vi "WFS Average Image Rolling.vi"(8 "error in (no error)":errorcluster {"code" format="%.0x"}, 9 "Reset":i32 format="%.0g", 10 "Average Count":i32 format="%.0g", 11 "instrument handle":refnum<visa-resource-name>) -> (0 "error out":errorcluster {"code" format="%.0x"}, 3 "instrument handle out":refnum<visa-resource-name>)   [LabVIEW 2020]
doc: "This VI generates a rolling averaged image based on all previously entered camera images in ImageBuf. The VI returns after each call and the averaged image is returned in ImageBuf and also stored in ImageBufAveraged.\n\nThe new rolling averaged image is calculated pixel by pixel according to the formula:\n(AverageCount - 1) * ImageBufAvg + ImageBuf) / AverageCount\n\nNote:\nAs soon as the image size is changed by VI ConfigureCam the averaging process is re-started.\nThis VI is not available in Highspeed Mode!"
uses:
  WFS_32.dll
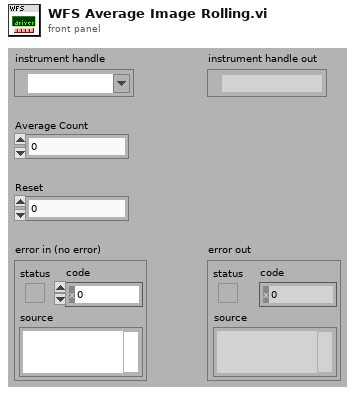
[diagram p1: front panel]
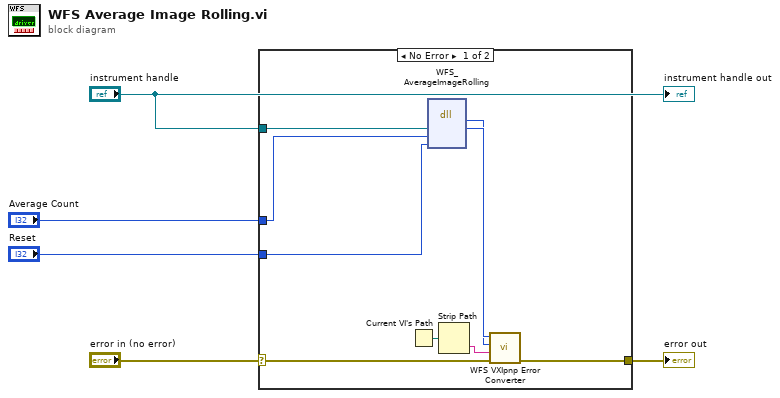
[diagram p0: block diagram]
diagram:
  n1 = case shown="No Error" "error in (no error)" {
    selector: "error in (no error)" -> [w9 w15]
    tunnel: [w8 w15] -> w5
    tunnel: "instrument handle" -> [w13 _]
    tunnel: "Average Count" -> [w7 _]
    tunnel: "Reset" -> [w6 _]
    frame No Error {
      n2 = Current VI's Path() -> (path=w14:path)
      n3 = dll-call lib="WFS_*.*" fn="WFS_AverageImageRolling"("Instrument Handle"=w13, "Average Count"=w7, "Reset"=w6) -> (w11:i32, "Instrument Handle"=w12:u32)  [unwired: 5 in, 2 out]
      n4 = Strip Path(path=w14) -> (name=w10:string)  [unwired: 1 out]
      n5 = call "WFS VXIpnp Error Converter.vi"("error in (no error)"=w9, "Name Of VI (\"\")"=w10, "CVI Error Code (0)"=w11, "instrument handle"=w12) -> ("error out"=w8:errorcluster)  [unwired: 6 in, 1 out]
    }
    frame Error {
    }
  }
  "error out" <- w5
  "instrument handle out" <- "instrument handle"
